vi "RSZVB Get Noise Figure LO Oscillator.vi"(8 "error in (no error)":errorcluster {"code" format="%.0x"}, 10 "Channel (1)":i32=1, 11 "VISA session":refnum<visa-resource-name>) -> (0 "error out":errorcluster {"code" format="%.0x"}, 1 "LO Oscillator":bool, 3 "dup VISA session":refnum<visa-resource-name>)   [LabVIEW 2011]
doc: "This VI returns whether the analyzer assumes an ideal T0 source noise. \n\nNote(s):\n\n(1) This VI is available only with option R&S ZVAB-K30.\n\nRemote-control command(s):\n[SENSe<Ch>:]NFIGure:ISNoise?"
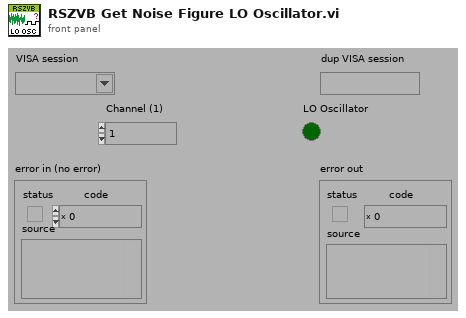
[diagram p1: front panel]
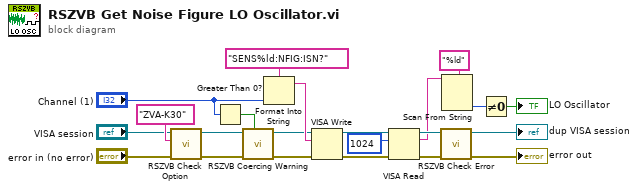
[diagram p0: block diagram]
diagram:
  n1 = call "RSZVB Check Option.vi"("error in (no error)"="error in (no error)", "Options"="ZVA-K30", "VISA session"="VISA session") -> ("error out"=w7:errorcluster, "dup VISA session"=w8:refnum<visa-resource-name>)  [unwired: 7 in]
  n2 = Greater Than 0?(x="Channel (1)") -> (x > 0?=w12:bool)
  n3 = call "RSZVB Coercing Warning.vi"("In Range?"=w12, "error in (no error)"=w7, "VISA session"=w8) -> ("error out"=w11:errorcluster, "dup VISA session"=w10:refnum<visa-resource-name>)  [unwired: 7 in]
  n4 = Format Into String(format string="SENS%ld:NFIG:ISN?", "Channel (1)") -> (resulting string=w13:string)  [unwired: 2 in, 1 out]
  n5 = VISA Write(VISA resource name=w10, write buffer=w13, error in (no error)=w11) -> (VISA resource name out=w22:refnum<visa-resource-name>, error out=w21:errorcluster)  [unwired: 1 out]
  n6 = VISA Read(VISA resource name=w22, byte count=u32 1024 ("byte count (0)"), error in (no error)=w21) -> (VISA resource name out=w19:refnum<visa-resource-name>, read buffer=w15:string, error out=w20:errorcluster)  [unwired: 1 out]
  n7 = call "RSZVB Check Error.vi"("error in (no error)"=w20, "VISA session"=w19) -> ("error out"=→"error out":errorcluster, "dup VISA session"=→"dup VISA session":refnum<visa-resource-name>)  [unwired: 8 in]
  n8 = Scan From String(format string="%ld", input string=w15) -> (output 1=w16:i32)  [unwired: 3 in, 3 out]
  n9 = Not Equal To 0?(x=w16) -> (x != 0?=→"LO Oscillator":bool)
